vi "BristolExample.vi"() -> ()   [LabVIEW 2014]
uses:
  RcvMsgType.ctl
  GlobalVars.vi
panel:
  out "Error Code":u32
  out "Prev Units":u32
  in  "Units":u32(ring) items=["nm", "GHz", "cm-1"]
  in  "Stop AutoScan Button":bool
  out "AutoScan Data":dbl=9.99 format="%.8f"
  in  "AutoScan Button":bool
  out "RxMsgCnt":u32
  in  "Rcv Msg Type":T1={"ID"=135, "Chksum"=123, "Unused"=0, "Length"=0, "Seq No"=0, "Msg Data"=[]}
  in  "Port":refnum<visa-resource-name>="COM1"
  in  "Exit  Button":bool
  out "Lambda Data":dbl=999.99999 format="%.5p"
  in  "Get Lambda Button":bool
  in  "Close Button":bool
  out "Connected":bool
  in  "Open Button":bool
  # "nm"
  # "Example Application Ver. 1.1"
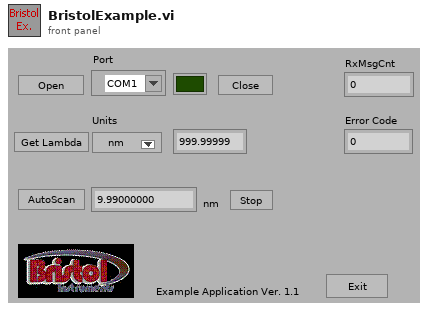
[diagram p1: front panel]
types:
  T1 = typedef "RcvMsgType.ctl" = cluster{"ID":u8, "Chksum":u16, "Unused":u16, "Length":u16, "Seq No":u8, "Msg Data":u8[]}
  T2 = typedef "Queue RefNum" = refnum<k1>
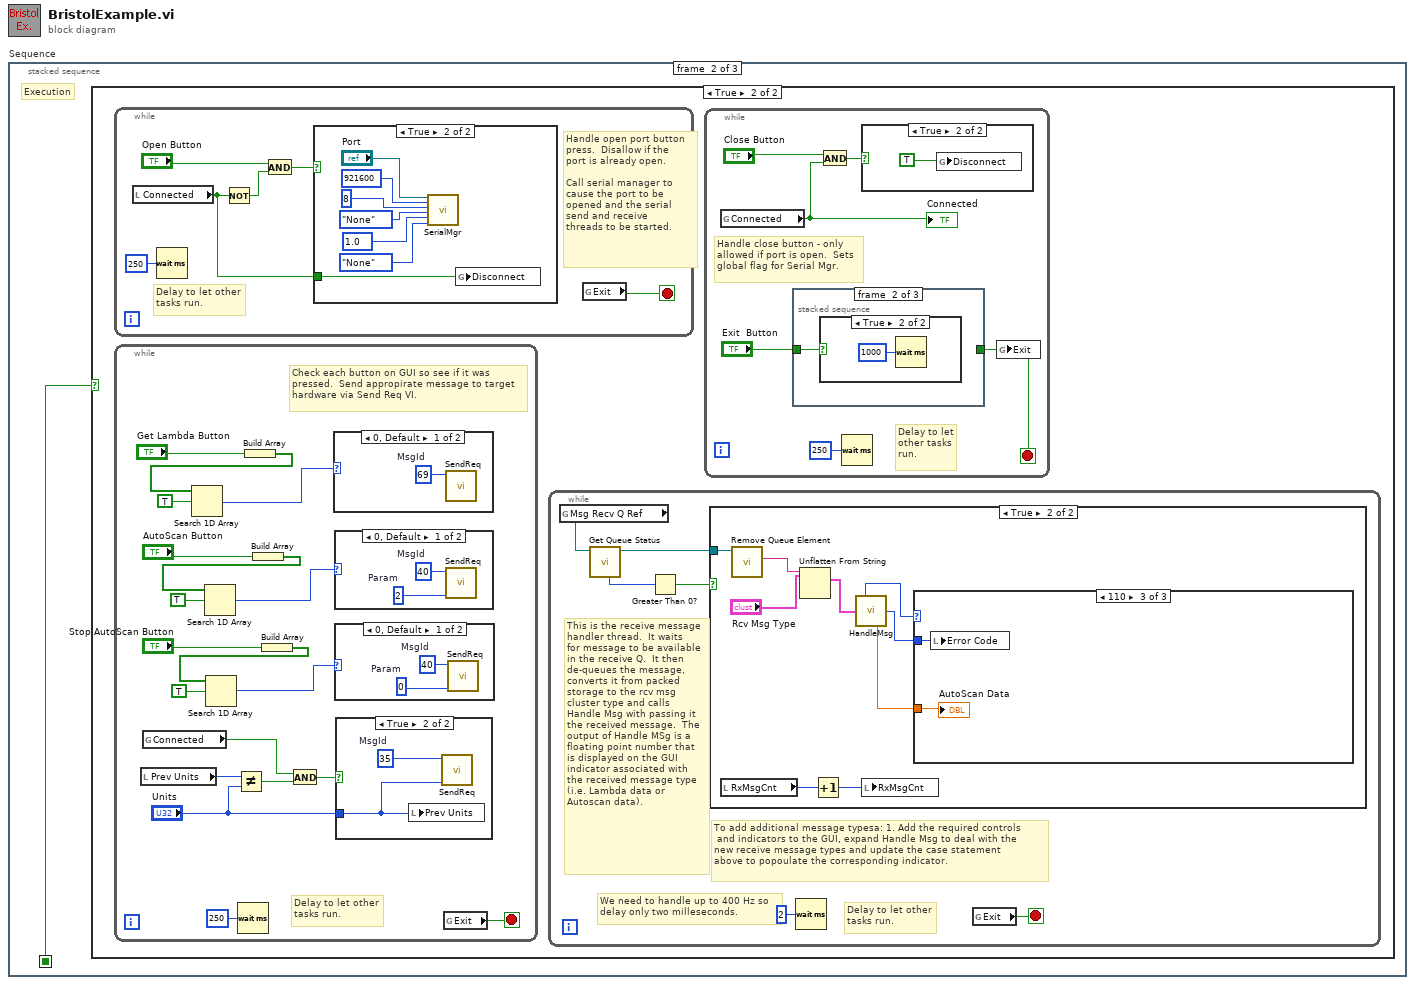
[diagram p0: block diagram]
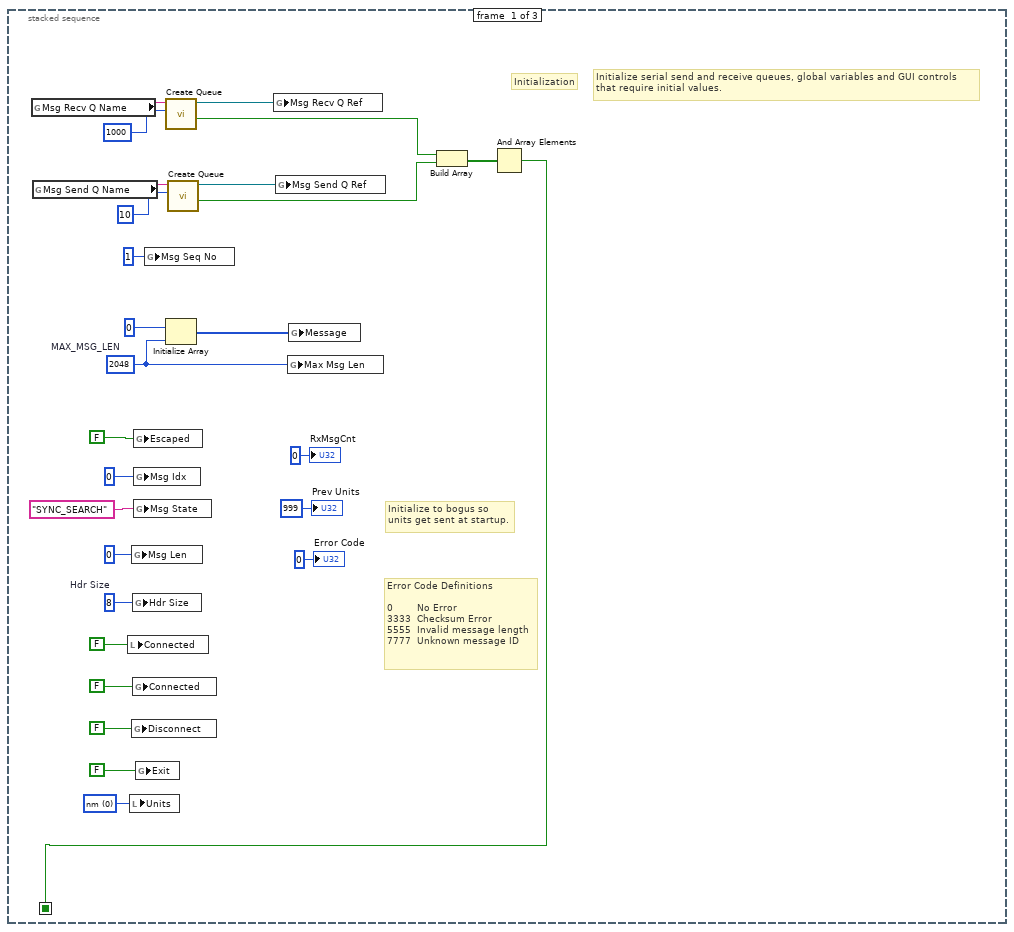
[diagram p2: hidden frame]
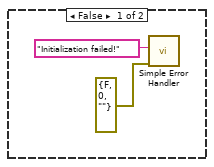
[diagram p3: hidden frame]
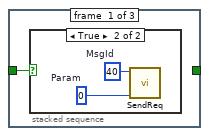
[diagram p8: hidden frame]
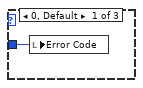
[diagram p15: hidden frame]
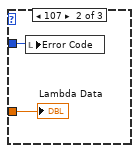
[diagram p16: hidden frame]
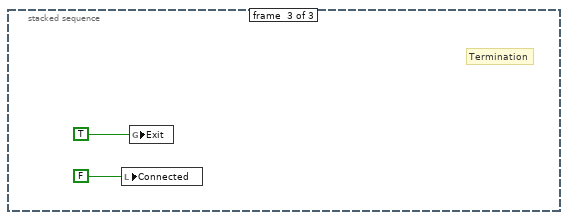
[diagram p17: hidden frame]
diagram:
  n1 = stacked-sequence "Sequence" {
    seq-local: [w4 _ _] -> [_ w28 _]
    frame #0 {
      w3 = u8 0 items=["nm", "GHz", "cm-1"] ("Units")
      w19 = u8 8  # Hdr Size
      w20 = 2048  # MAX_MSG_LEN
      # "Error Code Definitions\n\n0        No Error\n3333  Checksum Error\n5555  Invalid message length\n7777  Unknown message ID"
      # "Initialize to bogus so\nunits get sent at startup."
      # "Initialize serial send and receive queues, global variables and GUI controls\nthat require initial values."
      # "Initialization"
      n2 = global read "GlobalVars.vi" "Msg Recv Q Name"() -> (w26:string)
      n3 = global read "GlobalVars.vi" "Msg Send Q Name"() -> (w16:string)
      n4 = local write "Connected"(FALSE ("Connected")) -> ()
      n5 = local write "Units"(w3) -> ()
      n6 = global write "GlobalVars.vi" "Msg Len"(u32 0 ("Msg Len")) -> ()
      n7 = global write "GlobalVars.vi" "Disconnect"(FALSE ("Disconnect")) -> ()
      n8 = global write "GlobalVars.vi" "Hdr Size"(w19) -> ()
      n9 = global write "GlobalVars.vi" "Connected"(FALSE ("Connected")) -> ()
      n10 = global write "GlobalVars.vi" "Escaped"(FALSE ("Escaped")) -> ()
      n11 = global write "GlobalVars.vi" "Msg Idx"(u32 0 ("Msg Idx")) -> ()
      n12 = global write "GlobalVars.vi" "Msg State"("SYNC_SEARCH" ("Msg State")) -> ()
      n13 = global write "GlobalVars.vi" "Exit"(FALSE ("Exit")) -> ()
      n14 = global write "GlobalVars.vi" "Msg Seq No"(u32 1 ("Msg Idx")) -> ()
      n15 = call <vilib>:"Create Queue.vi"("size (unbounded)"=1000, "name (unnamed)"=w26) -> ("created new"=w13:bool, "queue out"=w27:T2)  [unwired: 3 in, 1 out]
      n16 = Initialize Array "Initialize Array"(u8 0 ("Element Data"), w20) -> (w25:u8[])
      n17 = call <vilib>:"Create Queue.vi"("size (unbounded)"=10, "name (unnamed)"=w16) -> ("created new"=w14:bool, "queue out"=w17:T2)  [unwired: 3 in, 1 out]
      n18 = global write "GlobalVars.vi" "Msg Recv Q Ref"(w27) -> ()
      n19 = global write "GlobalVars.vi" "Msg Send Q Ref"(w17) -> ()
      n20 = global write "GlobalVars.vi" "Max Msg Len"(w20) -> ()
      n21 = global write "GlobalVars.vi" "Message"(w25) -> ()
      n22 = Build Array(w13, w14) -> (w12:bool[])
      n23 = And Array Elements(Boolean array=w12) -> (logical AND=w4:bool)
      "RxMsgCnt" <- u32 0 ("RxMsgCnt")
      "Prev Units" <- u32 999 ("Prev Units")
      "Error Code" <- u32 0 ("Error Code")
    }
    frame #1 {
      # "Execution"
      n24 = case shown="True" w28 {
        frame False {
          n25 = call <vilib>:"Simple Error Handler.vi"("error source (\" \")"="Initialization failed!" ("error source (\" \")"), "error in (no error)"=errorcluster {"status"=FALSE, "code"=0, "source"=""}) -> ()  [unwired: 3 in, 5 out]
        }
        frame True {
          n26 = while {
            stop <- w70 stop-if-true
            # "Delay to let other\ntasks run."
            # "Handle open port button\npress.  Disallow if the\nport is already open.\n\nCall serial manager to\ncause the port to be\nopened and the serial\nsend and receive\nthreads to be started."
            n27 = local read "Connected"() -> (w72:bool)
            n28 = Wait (ms)(milliseconds to wait=u32 250) -> ()  [unwired: 1 out]
            n29 = Not(x=w72) -> (.not. x?=w75:bool)
            n30 = And(x="Open Button", y=w75) -> (x .and. y?=w73:bool)
            n31 = case shown="True" w73 {
              tunnel: w72 -> [_ w76]
              frame False {
              }
              frame True {
                w78 = u16 10 items=["1.0"=10, "1.5"=15, "2.0"=20] ("stop bits (10: 1 bit)")
                n32 = call "SerialMgr.vi"("VISA Resource Name"="Port", "baud rate (921600)"=u32 921600, "data bits (8)"=u16 8, "parity (0:none)"=enum16{"None", "Odd", "Even", "Mark", "Space"}."None", "stop bits (10: 1 bit)"=w78, "flow control (0:None)"=enum16{"None", "XON/XOFF", "RTS/CTS"}."None") -> ()  [unwired: 14 in]
                n33 = global write "GlobalVars.vi" "Disconnect"(w76) -> ()
              }
            }
            n34 = global read "GlobalVars.vi" "Exit"() -> (w70:bool)
          }
          n35 = while {
            stop <- w39 stop-if-true
            # "Delay to let other\ntasks run."
            # "Check each button on GUI so see if it was\npressed.  Send appropirate message to target\nhardware via Send Req VI."
            n36 = local read "Prev Units"() -> (w36:u32)
            n37 = global read "GlobalVars.vi" "Connected"() -> (w33:bool)
            n38 = Not Equal?(x=w36, y="Units") -> (x != y?=w34:bool)
            n39 = Wait (ms)(milliseconds to wait=u32 250) -> ()  [unwired: 1 out]
            n40 = Build Array "Build Array"("Get Lambda Button") -> (w48:bool[])
            n41 = Search 1D Array(1D array=w48, element=TRUE) -> (index of element=w31:i32)  [unwired: 1 in]
            n42 = Build Array "Build Array"("AutoScan Button") -> (w47:bool[])
            n43 = Search 1D Array(1D array=w47, element=TRUE) -> (index of element=w45:i32)  [unwired: 1 in]
            n44 = Build Array "Build Array"("Stop AutoScan Button") -> (w44:bool[])
            n45 = Search 1D Array(1D array=w44, element=TRUE) -> (index of element=w37:i32)  [unwired: 1 in]
            n46 = And(x=w33, y=w34) -> (x .and. y?=w32:bool)
            n47 = case shown="0, Default" w31 {
              frame 0, Default {
                w56 = u8 69  # MsgId
                (unwired) u8 69  # MsgId
                n48 = call "SendReq.vi"("MsgId"=w56) -> ()  [unwired: 4 in]
              }
              frame -1 {
              }
            }
            n49 = case shown="0, Default" w45 {
              frame 0, Default {
                w54 = u32 2  # Param
                w55 = u8 40  # MsgId
                n50 = call "SendReq.vi"("Param"=w54, "MsgId"=w55) -> ()  [unwired: 3 in]
              }
              frame -1 {
              }
            }
            n51 = case shown="0, Default" w37 {
              frame 0, Default {
                w52 = u32 0  # Param
                w53 = u8 40  # MsgId
                n52 = call "SendReq.vi"("Param"=w52, "MsgId"=w53) -> ()  [unwired: 3 in]
              }
              frame -1 {
              }
            }
            n53 = case shown="True" w32 {
              tunnel: "Units" -> [_ w50]
              frame False {
              }
              frame True {
                w51 = u8 35  # MsgId
                n54 = local write "Prev Units"(w50) -> ()
                n55 = call "SendReq.vi"("Param"=w50, "MsgId"=w51) -> ()  [unwired: 3 in]
              }
            }
            n56 = global read "GlobalVars.vi" "Exit"() -> (w39:bool)
          }
          n57 = while {
            stop <- w88 stop-if-true
            # "Delay to let other\ntasks run."
            # "To add additional message typesa: 1. Add the required controls \n and indicators to the GUI, expand Handle Msg to deal with the\nnew receive message types and update the case statement\nabove to popoulate the corresponding indicator."
            # "This is the receive message\nhandler thread.  It waits\nfor message to be available\nin the receive Q.  It then\nde-queues the message,\nconverts it from packed\nstorage to the rcv msg\ncluster type and calls\nHandle Msg with passing it\nthe received message.  The\noutput of Handle MSg is a\nfloating point number that\nis displayed on the GUI\nindicator associated with\nthe received message type\n(i.e. Lambda data or\nAutoscan data)."
            # "We need to handle up to 400 Hz so\ndelay only two milleseconds."
            n58 = global read "GlobalVars.vi" "Msg Recv Q Ref"() -> (w87:T2)
            n59 = call <vilib>:"Get Queue Status.vi"("queue"=w87) -> ("queue out"=w84:T2, "# elements in queue"=w86:i32)  [unwired: 3 in, 6 out]
            n60 = Greater Than 0?(x=w86) -> (x > 0?=w85:bool)
            n61 = case shown="True" w85 {
              tunnel: w84 -> [_ w97]
              frame False {
              }
              frame True {
                n62 = local read "RxMsgCnt"() -> (w93:u32)
                n63 = call <vilib>:"Remove Queue Element.vi"("queue"=w97) -> ("queue element"=w96:string)  [unwired: 5 in, 3 out]
                n64 = Unflatten From String(type="Rcv Msg Type", binary string=w96) -> (value=w94:T1)  [unwired: 3 in, 2 out]
                n65 = Increment(x=w93) -> (x+1=w92:u32)
                n66 = call "HandleMsg.vi"("Rcv Msg Type"=w94) -> ("ID"=w91:u8, "Uint32"=w89:u32, "Double 1"=w90:dbl)  [unwired: 5 in, 7 out]
                n67 = local write "RxMsgCnt"(w92) -> ()
                n68 = case shown="110" w91 {
                  tunnel: w90 -> [_ w100 w102]
                  tunnel: w89 -> [w98 w99 w101]
                  frame 0, Default {
                    n69 = local write "Error Code"(w98) -> ()
                  }
                  frame 107 {
                    n70 = local write "Error Code"(w99) -> ()
                    "Lambda Data" <- w100
                  }
                  frame 110 {
                    n71 = local write "Error Code"(w101) -> ()
                    "AutoScan Data" <- w102
                  }
                }
              }
            }
            n72 = Wait (ms)(milliseconds to wait=u32 2) -> ()  [unwired: 1 out]
            n73 = global read "GlobalVars.vi" "Exit"() -> (w88:bool)
          }
          n74 = while {
            stop <- w57 stop-if-true
            # "Delay to let\nother tasks\nrun."
            # "Handle close button - only\nallowed if port is open.  Sets\nglobal flag for Serial Mgr."
            n75 = global read "GlobalVars.vi" "Connected"() -> (w60:bool)
            "Connected" <- w60
            n76 = stacked-sequence {
              tunnel: "Exit  Button" -> [w63 w66 w68]
              tunnel: [_ _ w68] -> w57
              frame #0 {
                n77 = case shown="True" w63 {
                  frame False {
                  }
                  frame True {
                    w64 = u32 0  # Param
                    w65 = u8 40  # MsgId
                    n78 = call "SendReq.vi"("Param"=w64, "MsgId"=w65) -> ()  [unwired: 3 in]
                  }
                }
              }
              frame #1 {
                n79 = case shown="True" w66 {
                  frame False {
                  }
                  frame True {
                    n80 = Wait (ms)(milliseconds to wait=u32 1000) -> ()  [unwired: 1 out]
                  }
                }
              }
              frame #2 {
              }
            }
            n81 = And(x="Close Button", y=w60) -> (x .and. y?=w59:bool)
            n82 = Wait (ms)(milliseconds to wait=u32 250) -> ()  [unwired: 1 out]
            n83 = case shown="True" w59 {
              frame False {
              }
              frame True {
                n84 = global write "GlobalVars.vi" "Disconnect"(TRUE ("Connected")) -> ()
              }
            }
            n85 = global write "GlobalVars.vi" "Exit"(w57) -> ()
          }
        }
      }
    }
    frame #2 {
      # "Termination"
      n86 = local write "Connected"(FALSE ("Connected")) -> ()
      n87 = global write "GlobalVars.vi" "Exit"(TRUE ("Exit")) -> ()
    }
  }
